vi "Initialize.vi"(0 "Waveform in":refnum<class "Waveform.lvclass">, 1 "Filter in":refnum<class "Filter.lvclass">, 5 "Level in":refnum<class "Level.lvclass">, 7 "Fs (Hz)":dbl, 9 "Npts":i32, 11 "error in (no error)":errorcluster, 13 "Channel Name":string) -> (3 "Filter out":refnum<class "Filter.lvclass">, 4 "Waveform out":refnum<class "Waveform.lvclass">, 6 "Level out":refnum<class "Level.lvclass">, 15 "error out":errorcluster)   [LabVIEW 2015, in "Waveform.lvclass"]
uses:
  Waveform.lvclass
  Level/Level.lvclass
  Filter/Filter.lvclass
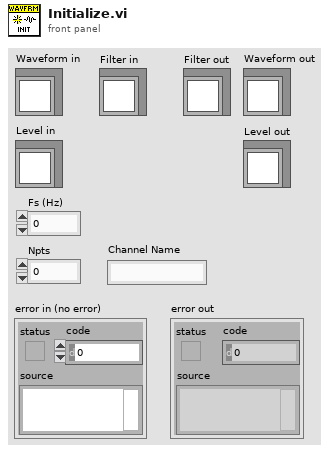
[diagram p1: front panel]
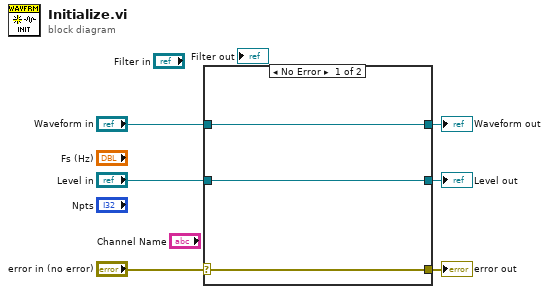
[diagram p0: block diagram]
diagram:
  n1 = case shown="No Error" "error in (no error)" {
    selector: "error in (no error)" -> [w8 w12]
    tunnel: [w8 w12] -> w5
    tunnel: [w9 w11] -> w3
    tunnel: "Waveform in" -> [w9 w11]
    tunnel: "Level in" -> [w7 w10]
    tunnel: [w7 w10] -> w1
    frame No Error {
    }
    frame Error {
    }
  }
  "error out" <- w5
  "Waveform out" <- w3
  "Level out" <- w1
